vi "GEA3 EMV Draw Trigger Development.vi"() -> ()   [LabVIEW 2016]
uses:
  type defs/ERD Write Data In.ctl
  type defs/Data Type.ctl
  Type Definitions/GEA3 HEWH ERD Data.ctl
  Type Definitions/GEA3 HEWH Mixing Valve.ctl
  Users/220038920/Desktop/GEA3 Toolkit/LabVIEW GEA3 Rev2 API Toolkit LV2016/Water Heating Specific/Type Definitions/GEA3 HEWH Personality.ctl
  <vilib>/Utility/error.llb/whitespace.ctl
  library/GEA2_Toolkit.lvlib
panel:
  in  "Board ID":string="DN03WH1F"
  in  "Reset Control Counter":bool
  in  "Update Personality":bool
  in  "Personality":T1
  in  "Update Ki Qbits":bool
  in  "Ki Qbits Value":i32=5
  in  "Ki Gain Value":i32=1
  in  "Update Ki Gain":bool
  in  "Update Kp Qbits":bool
  in  "Kp Qbits Value":i32=5
  in  "Update Kp Gain":bool
  in  "Kp Gain Value":i32=100
  in  "Update Capacity":bool
  in  "Capacity Setting":string(combo)
  in  "EMV MANUAL MODE (0x400D)":bool
  in  "Park Position Value":i32=250
  in  "Park Position":bool
  out "Step Position":i16(graph)
  out "T7 Flow Dectection/ERD Send":bool
  in  "Use MIN":bool=TRUE
  out "T7":dbl(graph)
  out "T6":dbl(graph)
  out "Flow Detect":string[][](array[string])
  out "Cycles":i32
  out "ERD Data":T2
  out "Raw Data Out":string
  in  "ERD Write Data In":T4 {"ERD Number" format="%.0x"}
  in  "Send?":bool
  in  "stop":bool
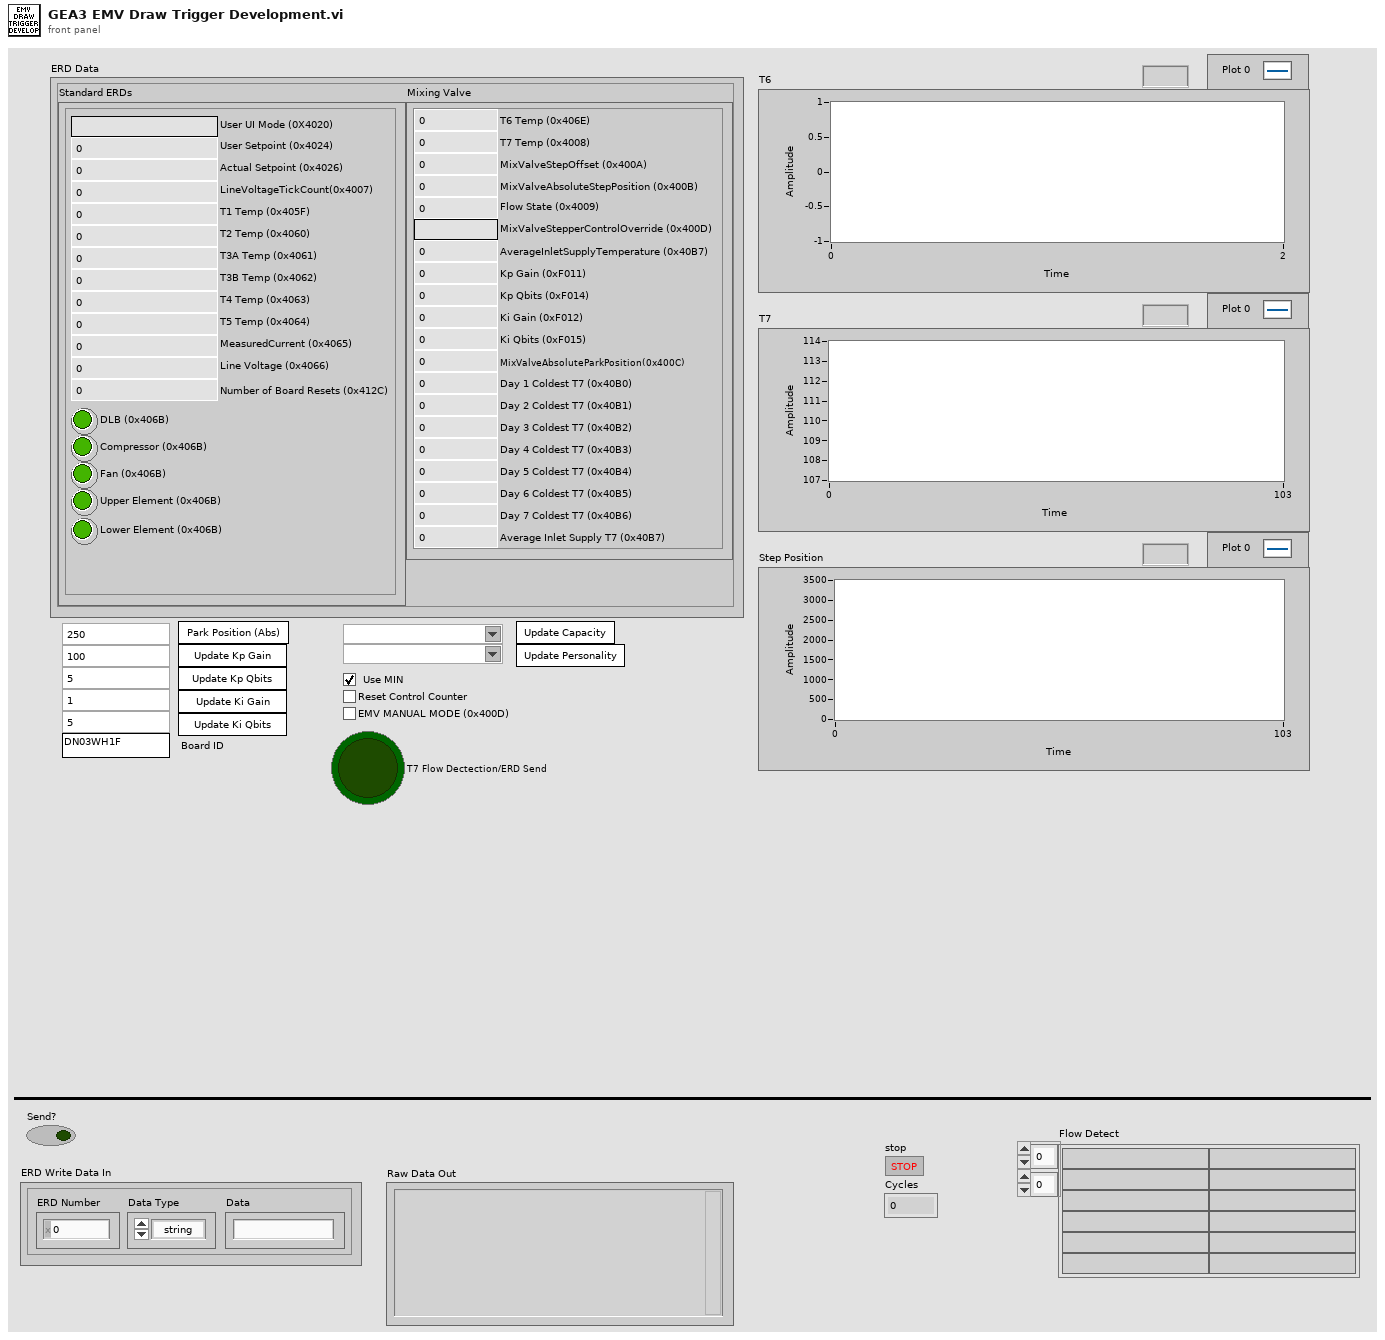
[diagram p1: front panel]
types:
  T1 = typedef "GEA3 HEWH Personality.ctl" = string
  T2 = typedef "GEA3 HEWH ERD Data.ctl" = cluster{"Mixing Valve":T3, "Standard ERDs":cluster{"User UI Mode (0X4020)":string, "User Setpoint (0x4024)":u16, "Actual Setpoint (0x4026)":u16, "DLB (0x406B)":bool, "Compressor (0x406B)":bool, "Lower Element (0x406B)":bool, "Upper Element (0x406B)":bool, "Fan (0x406B)":bool, "T1 Temp (0x405F)":dbl, "T2 Temp (0x4060)":dbl, "T3A Temp (0x4061)":dbl, "T3B Temp (0x4062)":dbl, "T4 Temp (0x4063)":dbl, "T5 Temp (0x4064)":dbl, "Line Voltage (0x4066)":dbl, "MeasuredCurrent (0x4065)":dbl, "LineVoltageTickCount(0x4007)":u16, "Number of Board Resets (0x412C)":u16}}
  T3 = typedef "GEA3 HEWH Mixing Valve.ctl" = cluster{"T7 Temp (0x4008)":dbl, "MixValveStepOffset (0x400A)":i16, "MixValveAbsoluteStepPosition (0x400B)":i16, "Flow State (0x4009)":u8, "MixValveStepperControlOverride (0x400D)":string, "AverageInletSupplyTemperature (0x40B7)":dbl, "T6 Temp (0x406E)":dbl, "Kp Gain (0xF011)":u16, "Kp Qbits (0xF014)":u16, "Ki Gain (0xF012)":u16, "Ki Qbits (0xF015)":u16, "MixValveAbsoluteParkPosition(0x400C)":i16, "Day 2 Coldest T7 (0x40B1)":dbl, "Day 1 Coldest T7 (0x40B0)":dbl, "Day 4 Coldest T7 (0x40B3)":dbl, "Day 3 Coldest T7 (0x40B2)":dbl, "Day 6 Coldest T7 (0x40B5)":dbl, "Day 5 Coldest T7 (0x40B4)":dbl, "Average Inlet Supply T7 (0x40B7)":dbl, "Day 7 Coldest T7 (0x40B6)":dbl}
  T4 = typedef "GEA2_Toolkit.lvlib/ERD Write Data In.ctl" = cluster{"ERD Number":u16, "Data Type":T5, "Data":string}
  T5 = typedef "GEA2_Toolkit.lvlib/Data Type.ctl" = enum16{"string", "boolean", "uint8_t", "uint16_t", "uint32_t", "uint64_t", "int8_t", "int16_t", "int32_t", "int64_t"}
  T6 = typedef "whitespace.ctl" = u16
  T7 = typedef "GEA2_Toolkit.lvlib/Source_Destination.ctl" = cluster{"Source":u8, "Destination":u8}
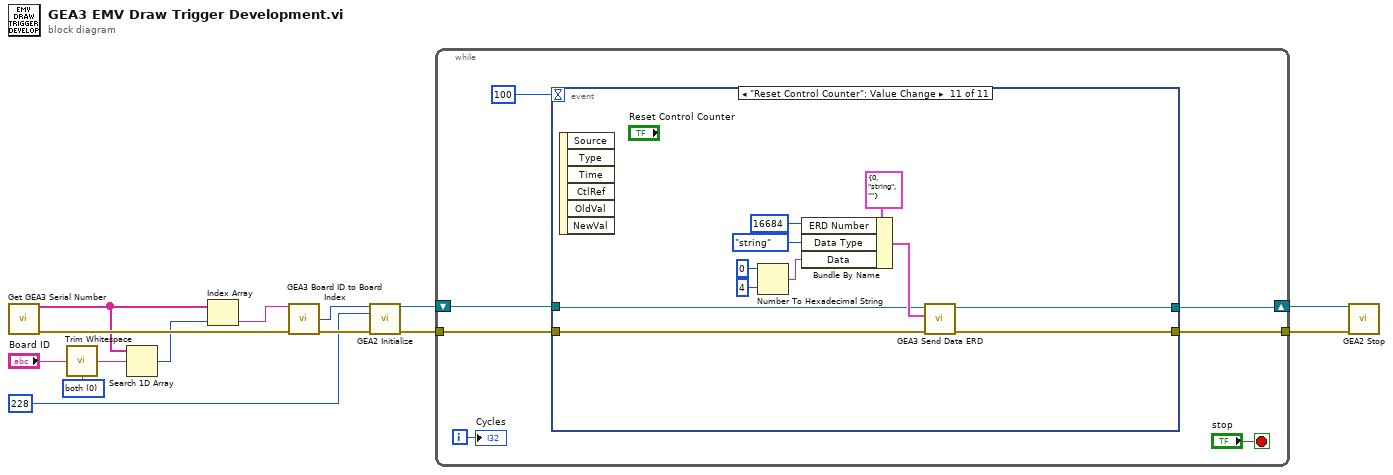
[diagram p0: block diagram]
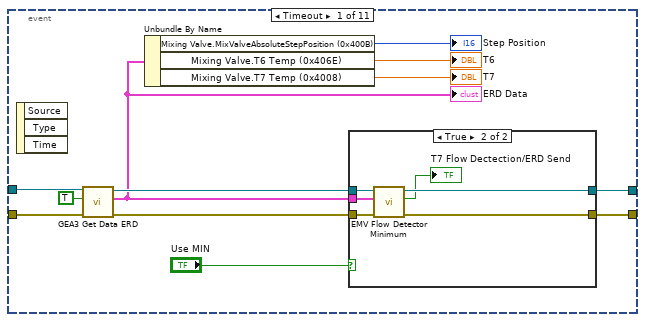
[diagram p2: hidden frame]
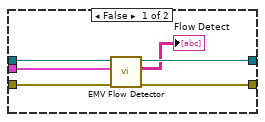
[diagram p3: hidden frame]
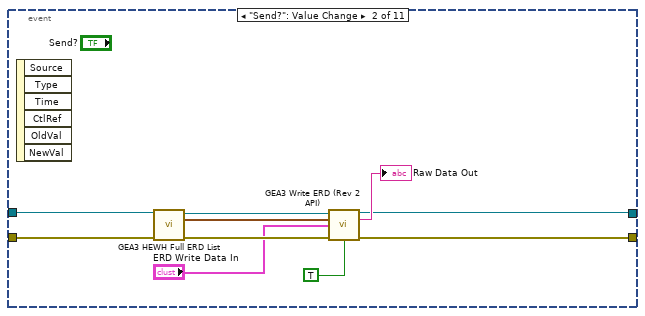
[diagram p4: hidden frame]
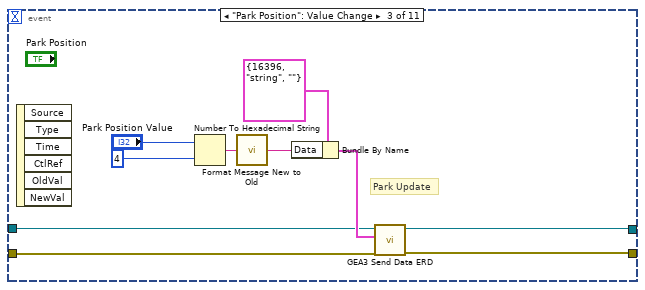
[diagram p5: hidden frame]
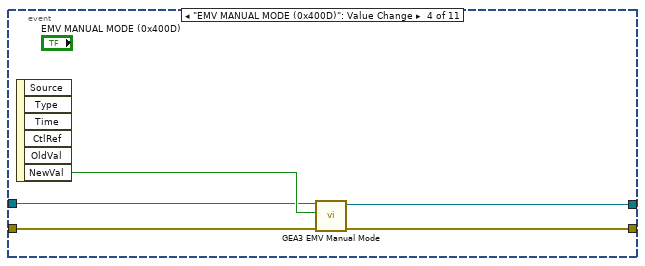
[diagram p6: hidden frame]
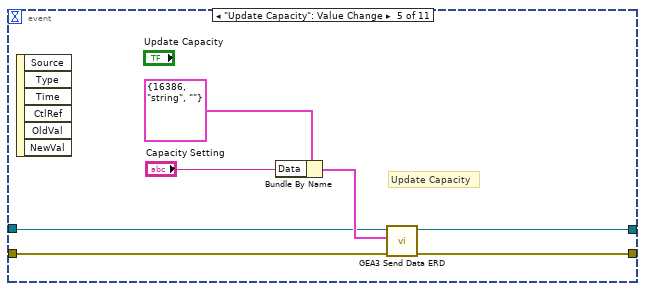
[diagram p7: hidden frame]
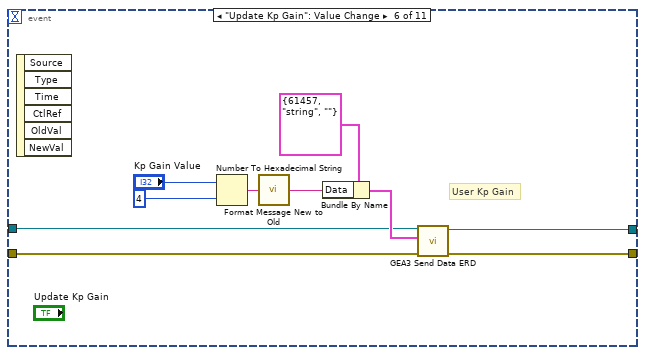
[diagram p8: hidden frame]
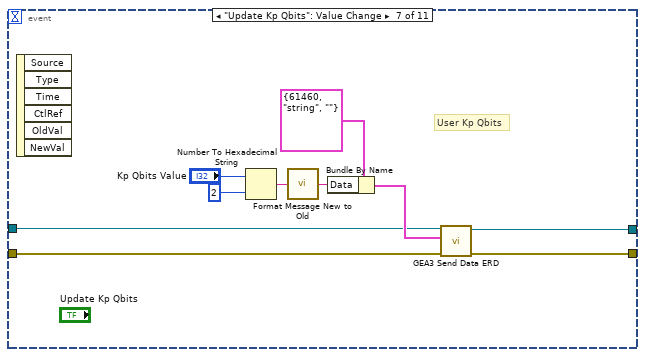
[diagram p9: hidden frame]
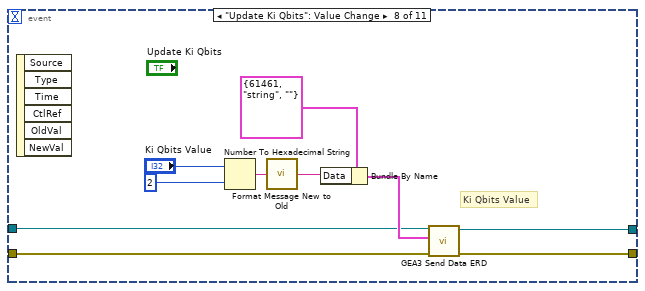
[diagram p10: hidden frame]
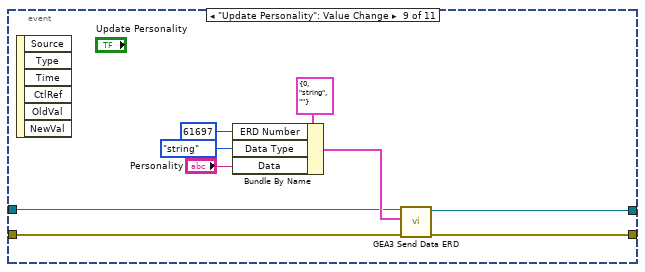
[diagram p11: hidden frame]
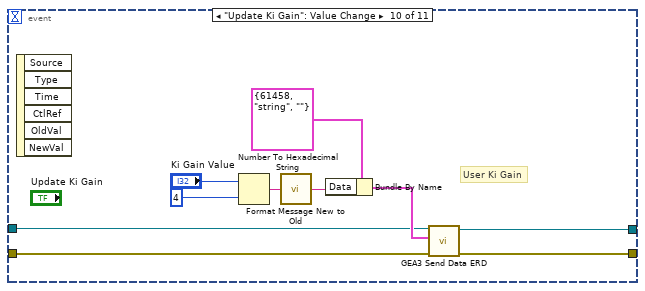
[diagram p12: hidden frame]
diagram:
  w1 = T6 0 items=["both", "start of string", "end of string"] ("location (both)")
  n1 = call "Get GEA3 Serial Number.vi"() -> ("GEA3 Serial Numbers"=w5:string[], "Error Out"=w11:errorcluster)  [unwired: 14 in]
  n2 = call <vilib>:"Trim Whitespace.vi"("string"="Board ID", "location (both)"=w1) -> ("trimmed string"=w2:string)
  n3 = Search 1D Array(1D array=w5, element=w2) -> (index of element=w6:i32)  [unwired: 1 in]
  n4 = Index Array(array=w5, index=w6) -> (element=w4:string)
  n5 = call "GEA3 Board ID to Board Index.vi"("GEA3 Serial Number"=w4, "Error In"=w11) -> ("Board Index"=w12:i32, "Error Out"=w13:errorcluster)  [unwired: 9 in, 3 out]
  n6 = call "GEA2 Initialize.vi"("Board Index"=w12, "Source Address"=u8 228, "error in"=w13) -> ("GEA2 Reference Out"=w8:refnum<k24>, "error out"=w9:errorcluster)  [unwired: 10 in, 1 out]
  n7 = while {
    shift-right: [w17] -> w14
    shift-left: w8 -> [w19]
    tunnel: w9 -> [w20]
    tunnel: [w18] -> w10
    i -> [w16]
    stop <- "stop" stop-if-true
    n8 = event shown="[10] \"Reset Control Counter\": Value Change" {
      selector: _ -> [_ _ _ _ _ _ _ _ _ _ _]
      dyn-events: _ -> [_ _ _ _ _ _ _ _ _ _ _]
      timeout: u32 100 ("millisecond multiple") -> [_ _ _ _ _ _ _ _ _ _ _]
      tunnel: w20 -> [w33 w50 w59 w70 w71 w81 w91 w101 w110 w120 w130]
      tunnel: w19 -> [w32 w47 w57 w68 w72 w80 w89 w98 w109 w119 w129]
      tunnel: [w29 w49 w58 w67 w74 w78 w90 w100 w111 w117 w127] -> w18
      tunnel: [w27 w48 w56 w66 w73 w79 w88 w99 w108 w118 w128] -> w17
      event Timeout {
        n9 = event-data() -> ()  [unwired: 1 in, 3 out]
        n10 = call "GEA3 Get Data ERD.vi"("error in (no error)"=w33, "Enable EMV List"=TRUE, ".NET Refnum in"=w32) -> ("error out"=w30:errorcluster, "ERD Data  2"=w26:T2, ".NET Refnum out"=w28:refnum<k24>)  [unwired: 5 in, 1 out]
        "ERD Data" <- w26
        n11 = Unbundle By Name(w26) -> ("Mixing Valve.MixValveAbsoluteStepPosition (0x400B)"=→"Step Position":i16, "Mixing Valve.T6 Temp (0x406E)"=→"T6":dbl, "Mixing Valve.T7 Temp (0x4008)"=→"T7":dbl)
        n12 = case shown="True" "Use MIN" {
          tunnel: w30 -> [w39 w45]
          tunnel: [w38 w44] -> w29
          tunnel: w28 -> [w37 w43]
          tunnel: [w36 w42] -> w27
          tunnel: w26 -> [w34 w41]
          frame False {
            n13 = call "EMV Flow Detector.vi"("error in (no error)"=w39, "ERD Data"=w34, ".NET Refnum in"=w37) -> ("error out"=w38:errorcluster, "Flow Detect"=→"Flow Detect":string[][], ".NET Refnum out"=w36:refnum<k24>)  [unwired: 6 in]
          }
          frame True {
            n14 = call "EMV Flow Detector Minimum.vi"("error in (no error)"=w45, "ERD Data"=w41, ".NET Refnum in"=w43) -> ("error out"=w44:errorcluster, "T7 Flow Dectection"=→"T7 Flow Dectection/ERD Send":bool, ".NET Refnum out"=w42:refnum<k24>)  [unwired: 6 in]
          }
        }
      }
      event "Send?": Value Change {
        n15 = event-data() -> ()  [unwired: 1 in, 6 out]
        n16 = call "GEA3 HEWH Full ERD List.vi"("error in (no error)"=w50, "GEA2 Reference In"=w47) -> ("error out"=w53:errorcluster, "GEA Inputs"=w52:T7, "GEA2 Reference Out"=w51:refnum<k24>)  [unwired: 5 in, 2 out]
        n17 = call "GEA3 Write ERD (Rev 2 API).vi"("GEA2 Reference In"=w51, "GEA Inputs"=w52, "ERD Write Data In"="ERD Write Data In", "Error In"=w53, "Verify ERD Response?"=TRUE) -> ("GEA2 Reference Out"=w48:refnum<k24>, "Raw Data Out"=→"Raw Data Out":string, "Error Out"=w49:errorcluster)  [unwired: 7 in, 1 out]
      }
      event "Park Position": Value Change {
        # "Park Update"
        n18 = event-data() -> ()  [unwired: 1 in, 6 out]
        n19 = Number To Hexadecimal String(1:i16 4 ("width (-)"), 2:"Park Position Value") -> (0:w62:string)
        n20 = call "Format Message New to Old.vi"("Raw Message In"=w62) -> ("Conv Message Out"=w60:string)  [unwired: 14 in]
        n21 = Bundle By Name(cluster=T4 {"ERD Number"=16396, "Data Type"=enum."string", "Data"=""} ("ERD Write Data In"), "Data"=w60) -> (w65:T4)
        n22 = call "GEA3 Send Data ERD.vi"("error in (no error)"=w59, "ERD Write Data In"=w65, ".NET Refnum in"=w57) -> ("error out"=w58:errorcluster, "GEA2 Reference Out"=w56:refnum<k24>)  [unwired: 5 in, 2 out]
      }
      event "EMV MANUAL MODE (0x400D)": Value Change {
        n23 = event-data() -> ("NewVal"=w69:bool)  [unwired: 1 in, 5 out]
        n24 = call "GEA3 EMV Manual Mode.vi"("error in (no error)"=w70, "Manual Mode?"=w69, ".NET Refnum in"=w68) -> ("error out"=w67:errorcluster, "GEA2 Reference Out"=w66:refnum<k24>)  [unwired: 7 in]
      }
      event "Update Capacity": Value Change {
        # "Update Capacity"
        n25 = event-data() -> ()  [unwired: 1 in, 6 out]
        n26 = Bundle By Name(cluster=T4 {"ERD Number"=16386, "Data Type"=enum."string", "Data"=""} ("ERD Write Data In"), "Data"="Capacity Setting") -> (w77:T4)
        n27 = call "GEA3 Send Data ERD.vi"("error in (no error)"=w71, "ERD Write Data In"=w77, ".NET Refnum in"=w72) -> ("error out"=w74:errorcluster, "GEA2 Reference Out"=w73:refnum<k24>)  [unwired: 5 in, 2 out]
      }
      event "Update Kp Gain": Value Change {
        # "User Kp Gain"
        n28 = event-data() -> ()  [unwired: 1 in, 6 out]
        n29 = Number To Hexadecimal String(1:i16 4 ("width (-)"), 2:"Kp Gain Value") -> (0:w84:string)
        n30 = call "Format Message New to Old.vi"("Raw Message In"=w84) -> ("Conv Message Out"=w82:string)  [unwired: 14 in]
        n31 = Bundle By Name(cluster=T4 {"ERD Number"=61457, "Data Type"=enum."string", "Data"=""} ("ERD Write Data In"), "Data"=w82) -> (w87:T4)
        n32 = call "GEA3 Send Data ERD.vi"("error in (no error)"=w81, "ERD Write Data In"=w87, ".NET Refnum in"=w80) -> ("error out"=w78:errorcluster, "GEA2 Reference Out"=w79:refnum<k24>)  [unwired: 5 in, 2 out]
      }
      event "Update Kp Qbits": Value Change {
        # "User Kp Qbits"
        n33 = event-data() -> ()  [unwired: 1 in, 6 out]
        n34 = Number To Hexadecimal String(1:i16 2 ("width (-)"), 2:"Kp Qbits Value") -> (0:w93:string)
        n35 = call "Format Message New to Old.vi"("Raw Message In"=w93) -> ("Conv Message Out"=w92:string)  [unwired: 14 in]
        n36 = Bundle By Name(cluster=T4 {"ERD Number"=61460, "Data Type"=enum."string", "Data"=""} ("ERD Write Data In"), "Data"=w92) -> (w97:T4)
        n37 = call "GEA3 Send Data ERD.vi"("error in (no error)"=w91, "ERD Write Data In"=w97, ".NET Refnum in"=w89) -> ("error out"=w90:errorcluster, "GEA2 Reference Out"=w88:refnum<k24>)  [unwired: 5 in, 2 out]
      }
      event "Update Ki Qbits": Value Change {
        # "Ki Qbits Value"
        n38 = event-data() -> ()  [unwired: 1 in, 6 out]
        n39 = Number To Hexadecimal String(1:i16 2 ("width (-)"), 2:"Ki Qbits Value") -> (0:w103:string)
        n40 = call "Format Message New to Old.vi"("Raw Message In"=w103) -> ("Conv Message Out"=w102:string)  [unwired: 14 in]
        n41 = Bundle By Name(cluster=T4 {"ERD Number"=61461, "Data Type"=enum."string", "Data"=""} ("ERD Write Data In"), "Data"=w102) -> (w107:T4)
        n42 = call "GEA3 Send Data ERD.vi"("error in (no error)"=w101, "ERD Write Data In"=w107, ".NET Refnum in"=w98) -> ("error out"=w100:errorcluster, "GEA2 Reference Out"=w99:refnum<k24>)  [unwired: 5 in, 2 out]
      }
      event "Update Personality": Value Change {
        n43 = event-data() -> ()  [unwired: 1 in, 6 out]
        n44 = Bundle By Name(cluster=T4 {"ERD Number"=0, "Data Type"=enum."string", "Data"=""} ("ERD Write Data In"), "ERD Number"=u16 61697, "Data Type"=Data_Type."string", "Data"="Personality") -> (w113:T4)
        n45 = call "GEA3 Send Data ERD.vi"("error in (no error)"=w110, "ERD Write Data In"=w113, ".NET Refnum in"=w109) -> ("error out"=w111:errorcluster, "GEA2 Reference Out"=w108:refnum<k24>)  [unwired: 5 in, 2 out]
      }
      event "Update Ki Gain": Value Change {
        # "User Ki Gain"
        n46 = event-data() -> ()  [unwired: 1 in, 6 out]
        n47 = Number To Hexadecimal String(1:i16 4 ("width (-)"), 2:"Ki Gain Value") -> (0:w122:string)
        n48 = call "Format Message New to Old.vi"("Raw Message In"=w122) -> ("Conv Message Out"=w121:string)  [unwired: 14 in]
        n49 = Bundle By Name(cluster=T4 {"ERD Number"=61458, "Data Type"=enum."string", "Data"=""} ("ERD Write Data In"), "Data"=w121) -> (w126:T4)
        n50 = call "GEA3 Send Data ERD.vi"("error in (no error)"=w120, "ERD Write Data In"=w126, ".NET Refnum in"=w119) -> ("error out"=w117:errorcluster, "GEA2 Reference Out"=w118:refnum<k24>)  [unwired: 5 in, 2 out]
      }
      event "Reset Control Counter": Value Change {
        n51 = event-data() -> ()  [unwired: 1 in, 6 out]
        n52 = Number To Hexadecimal String(1:i16 4 ("width (-)"), 2:0 ("number")) -> (0:w131:string)
        n53 = Bundle By Name(cluster=T4 {"ERD Number"=0, "Data Type"=enum."string", "Data"=""} ("ERD Write Data In"), "ERD Number"=u16 16684, "Data Type"=Data_Type."string", "Data"=w131) -> (w135:T4)
        n54 = call "GEA3 Send Data ERD.vi"("error in (no error)"=w130, "ERD Write Data In"=w135, ".NET Refnum in"=w129) -> ("error out"=w127:errorcluster, "GEA2 Reference Out"=w128:refnum<k24>)  [unwired: 5 in, 2 out]
      }
    }
    "Cycles" <- w16
  }
  n55 = call "GEA2 Stop.vi"("GEA2 Reference In"=w14, "Error In"=w10) -> ()  [unwired: 13 in, 1 out]
